vi "Reset.vi"(8 "error in (no error)":errorcluster, 11 "Tektronic in":refnum<class "Tektronic.lvclass">) -> (0 "error out":errorcluster, 3 "Tektronic out":refnum<class "Tektronic.lvclass">)   [LabVIEW 2020, in "Controlador.lvlib" / "Tektronic.lvclass"]
uses:
  Tektronic.lvclass
  Tektronic.lvclass/Tektronic.ctl
  <instrlib>/Tektronix TDS 200 1000 2000 Series/Tektronix TDS 200 1000 2000 Series.lvlib
  C:/GitClones/Osciloscope modules/Modulo_Cloneable_DQMH/Libraries/Controlador/Class/Osciloscope/Osciloscope.lvclass
  C:/GitClones/Osciloscope modules/Modulo_Cloneable_DQMH/Libraries/Controlador/Class/Tektronic/Tektronic.lvclass
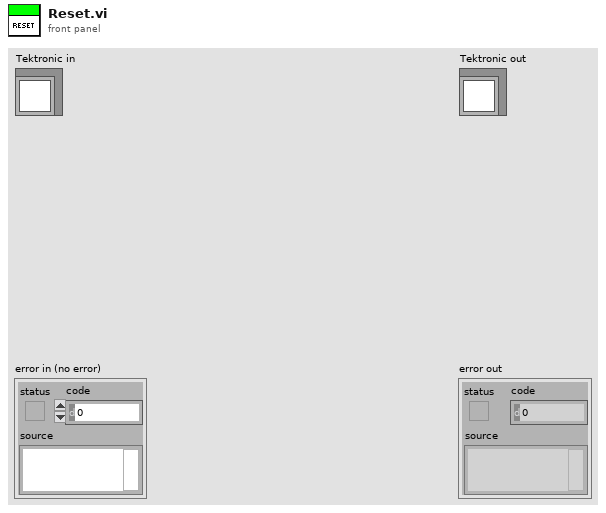
[diagram p1: front panel]
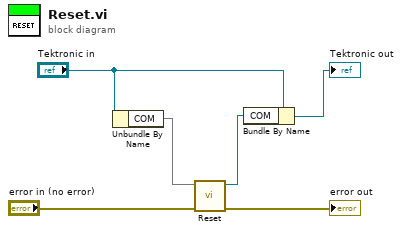
[diagram p0: block diagram]
diagram:
  n1 = Unbundle By Name("Tektronic in") -> ("COM"=w4)
  n2 = call <instrlib>:"Reset.vi"("error in (no error)"="error in (no error)", "VISA resource name"=w4) -> ("error out"=→"error out":errorcluster, "VISA resource name out"=w1:refnum<visa-resource-name>)  [unwired: 8 in]
  n3 = Bundle By Name(cluster="Tektronic in", "COM"=w1) -> (→"Tektronic out":refnum<class "Tektronic.lvclass">)
